vi "Treat Command.vi"(8 "error in (no error)":errorcluster, 11 "Channel in":refnum<class "Channel.lvclass">) -> (0 "error out":errorcluster, 3 "Channel out":refnum<class "Channel.lvclass">)   [LabVIEW 2018, in "Channel.lvclass"]
uses:
  Channel.lvclass
  Channel.lvclass/Channel.ctl
  TCS_ACS/TCS.lvclass/TCS.ctl
  Simulated_CCD_Camera/Simulated_CCD_Camera.lvclass/Simulated_CCD_Camera.ctl
  State Machine/State Machine.lvclass
  Simulated_CCD_Camera/Simulated_CCD_Camera.lvclass
  RxTx/RxTx.lvclass
  TCS_ACS/TCS.lvclass
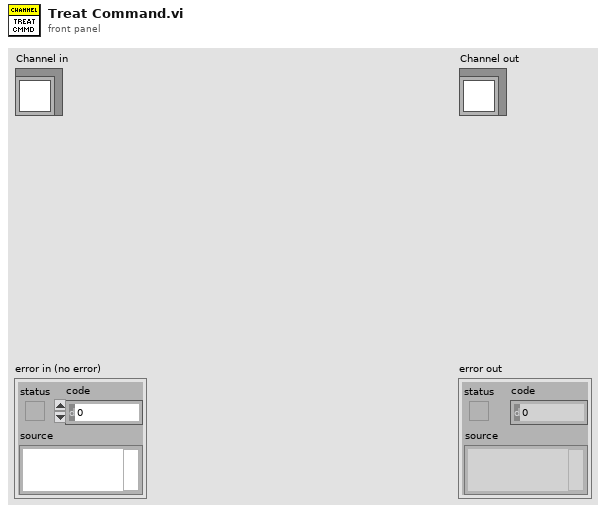
[diagram p1: front panel]
types:
  T1 = cluster{"CUBE_EXPOSURE_TIME":sgl, "CUBES_DONE":u16, "LAST_IMAGE_NAME":string, "DISK_SPACE":u16, "FRAMES_DONE":u16, "CCD_STATUS":string, "CURRENT_TEMPERATURE":i16, "TEMPERATURE_STATUS":string, "FRAME_EXPOSURE_TIME":dbl, "CCD_POWER_STATUS":bool, "SERIAL_NUMBER":u16, "ACQUIRING":bool}
  T2 = cluster{"COOLER_POWER_STATUS":u16, "TEMP":i32, "EXPTIME":sgl, "#FRAMES":u32, "#CUBES":u32}
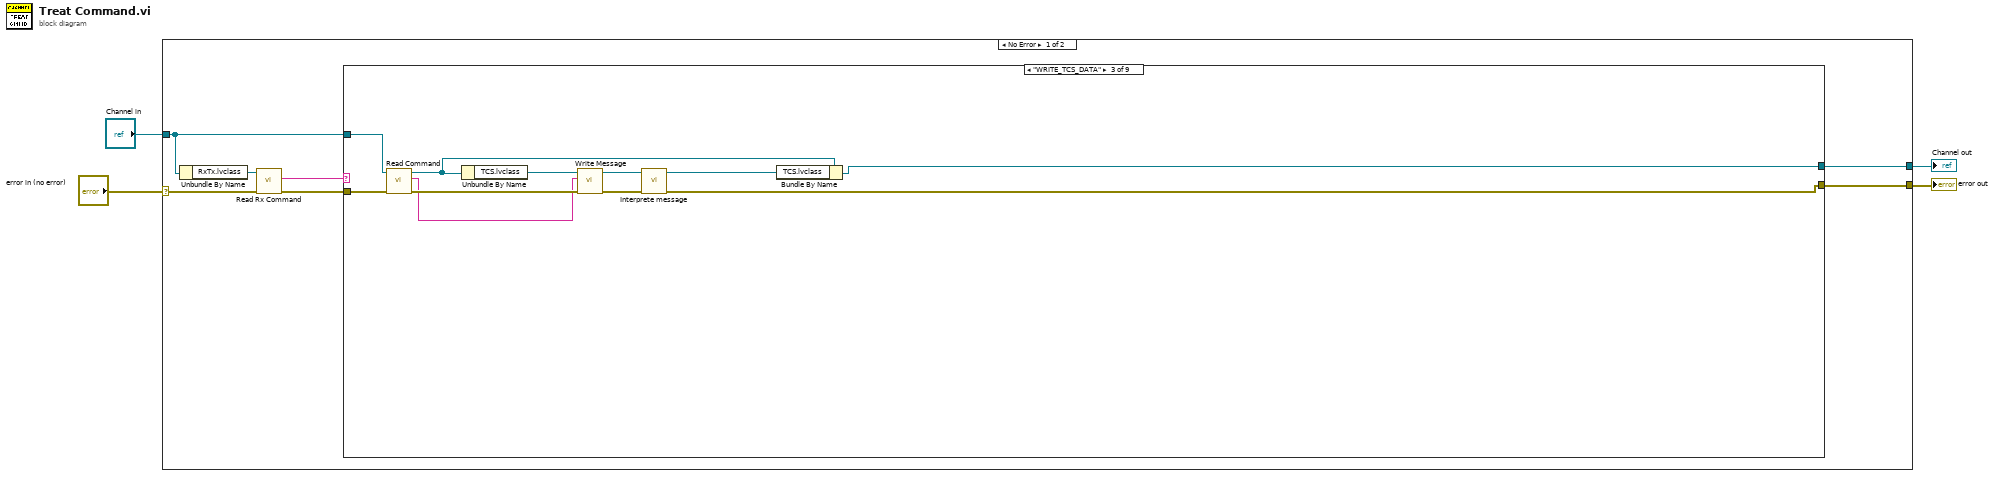
[diagram p0: block diagram]
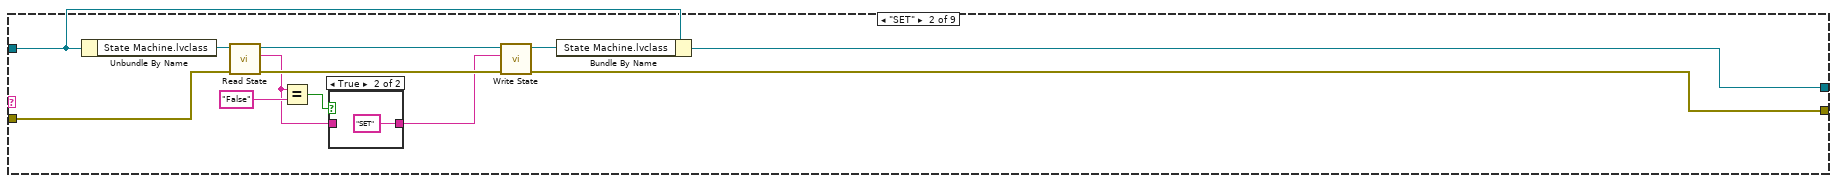
[diagram p3: hidden frame]
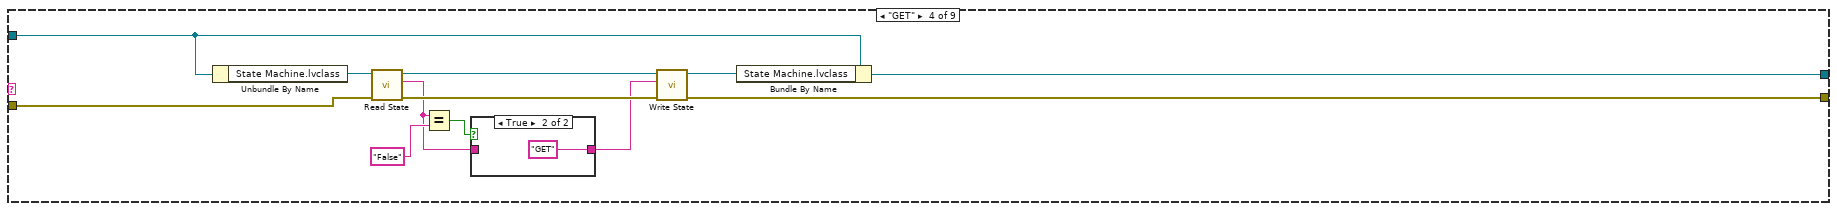
[diagram p5: hidden frame]
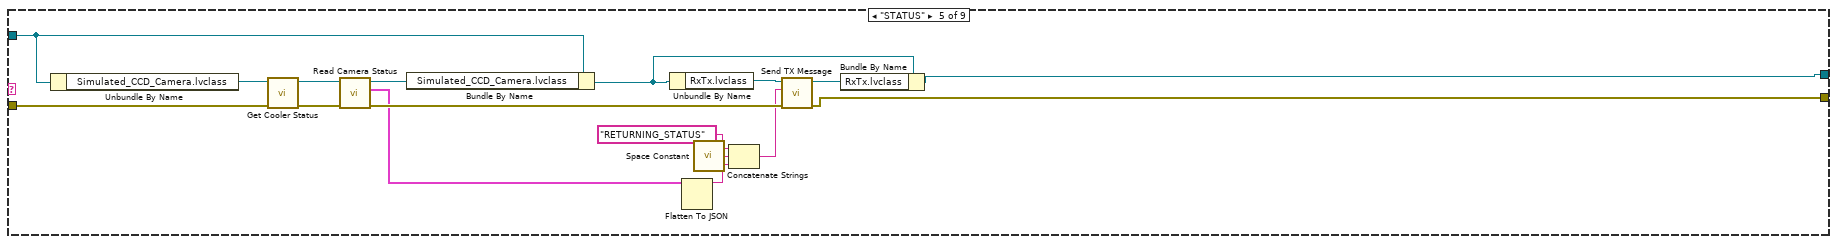
[diagram p7: hidden frame]
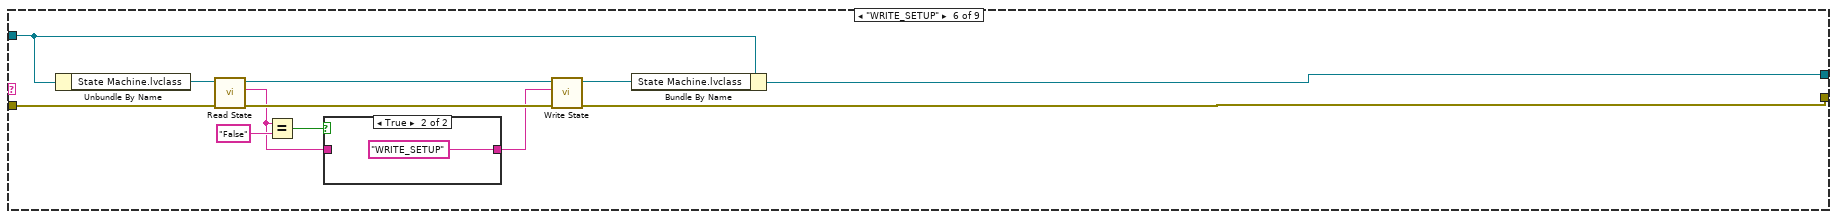
[diagram p8: hidden frame]
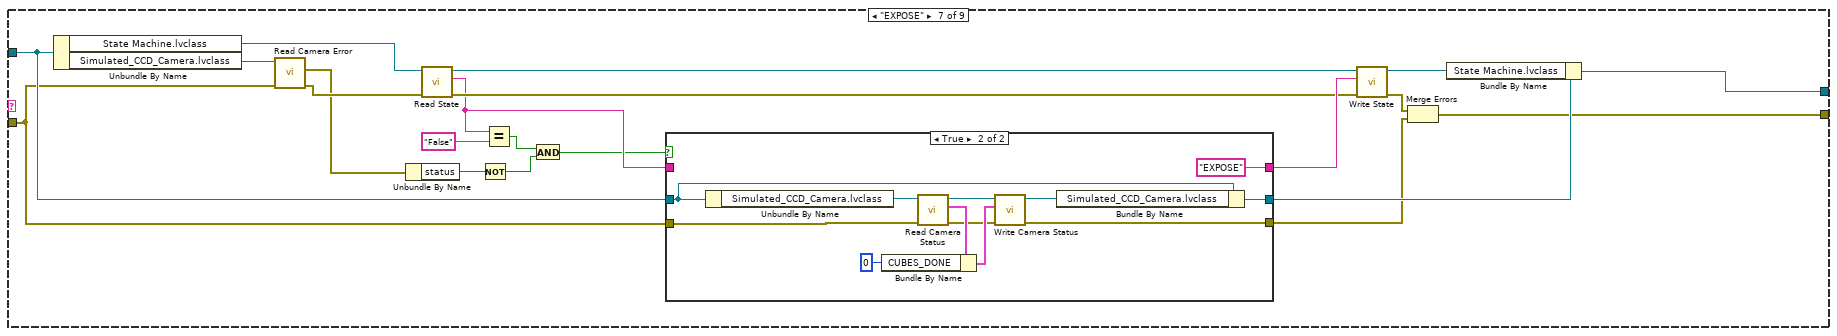
[diagram p10: hidden frame]
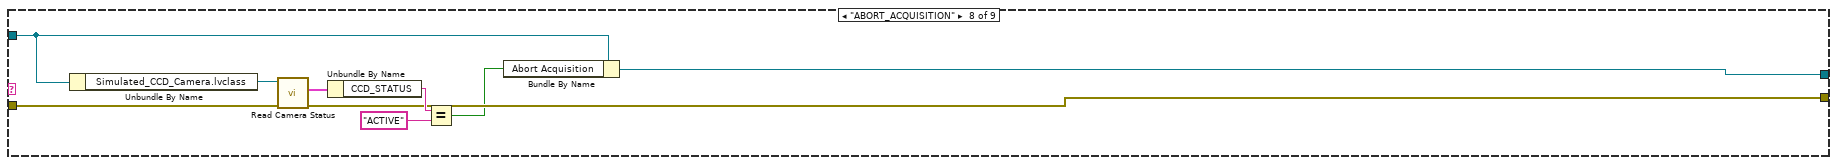
[diagram p12: hidden frame]
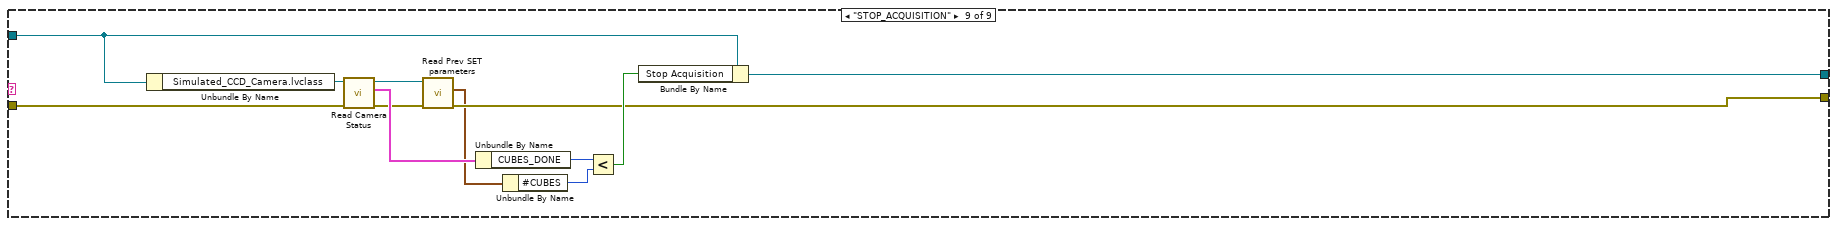
[diagram p13: hidden frame]
diagram:
  n1 = case shown="No Error" "error in (no error)" {
    selector: "error in (no error)" -> [w10 w142]
    tunnel: [w5 w142] -> w3
    tunnel: [w7 w141] -> w1
    tunnel: "Channel in" -> [w8 w141]
    frame No Error {
      n2 = Unbundle By Name(w8) -> ("RxTx.lvclass"=w11:refnum<class "RxTx.lvclass">)
      n3 = call "Read Rx Command.vi"("error in (no error)"=w10, "RxTx in"=w11) -> ("error out"=w6:errorcluster, "Rx Command"=w9:string)  [unwired: 7 in, 1 out]
      n4 = case shown="\"WRITE_TCS_DATA\"" w9 {
        tunnel: w8 -> [w13 w17 w37 w41 w69 w70 w98 w128 w138]
        tunnel: [w13 w14 w32 w40 w54 w76 w103 w127 w140] -> w7
        tunnel: w6 -> [w12 w16 w38 w42 w63 w74 w90 w122 w131]
        tunnel: [w12 w15 w28 w39 w53 w72 w96 w123 w134] -> w5
        frame "False", Default {
        }
        frame "SET" {
          n5 = Unbundle By Name(w17) -> ("State Machine.lvclass"=w23:refnum<class "State Machine.lvclass">)
          n6 = call-dynamic "Read State.vi"("error in (no error)"=w16, "State Machine in"=w23) -> ("error out"=w24:errorcluster, "State"=w19:string, "State Machine out"=w20:refnum<class "State Machine.lvclass">)  [unwired: 7 in]
          n7 = Equal?(x=w19, y="False") -> (x = y?=w18:bool)
          n8 = case shown="True" w18 {
            tunnel: [w26 "SET"] -> w22
            tunnel: w19 -> [w26 _]
            frame False {
            }
            frame True {
            }
          }
          n9 = call-dynamic "Write State.vi"("error in (no error)"=w24, "State"=w22, "State Machine in"=w20) -> ("error out"=w15:errorcluster, "State Machine out"=w25:refnum<class "State Machine.lvclass">)  [unwired: 7 in]
          n10 = Bundle By Name(cluster=w17, "State Machine.lvclass"=w25) -> (w14:refnum<class "Channel.lvclass">)
        }
        frame "WRITE_TCS_DATA" {
          n11 = call "Read Command.vi"("error in (no error)"=w38, "Channel in"=w37) -> ("error out"=w35:errorcluster, "Message"=w34:string, "Channel out"=w33:refnum<class "Channel.lvclass">)  [unwired: 7 in]
          n12 = Unbundle By Name(w33) -> ("TCS.lvclass"=w36:refnum<class "TCS.lvclass">)
          n13 = call "Write Message.vi"("error in (no error)"=w35, "Message"=w34, "TCS_ACS in"=w36) -> ("error out"=w29:errorcluster, "TCS_ACS out"=w31:refnum<class "TCS.lvclass">)  [unwired: 7 in]
          n14 = call "Interprete message.vi"("error in (no error)"=w29, "TCS_ACS in"=w31) -> ("error out"=w28:errorcluster, "TCS_ACS out"=w30:refnum<class "TCS.lvclass">)  [unwired: 8 in]
          n15 = Bundle By Name(cluster=w33, "TCS.lvclass"=w30) -> (w32:refnum<class "Channel.lvclass">)
        }
        frame "GET" {
          n16 = Unbundle By Name(w41) -> ("State Machine.lvclass"=w48:refnum<class "State Machine.lvclass">)
          n17 = call-dynamic "Read State.vi"("error in (no error)"=w42, "State Machine in"=w48) -> ("error out"=w49:errorcluster, "State"=w44:string, "State Machine out"=w45:refnum<class "State Machine.lvclass">)  [unwired: 7 in]
          n18 = Equal?(x=w44, y="False") -> (x = y?=w43:bool)
          n19 = case shown="True" w43 {
            tunnel: [w51 "GET"] -> w47
            tunnel: w44 -> [w51 _]
            frame False {
            }
            frame True {
            }
          }
          n20 = call-dynamic "Write State.vi"("error in (no error)"=w49, "State"=w47, "State Machine in"=w45) -> ("error out"=w39:errorcluster, "State Machine out"=w50:refnum<class "State Machine.lvclass">)  [unwired: 7 in]
          n21 = Bundle By Name(cluster=w41, "State Machine.lvclass"=w50) -> (w40:refnum<class "Channel.lvclass">)
        }
        frame "STATUS" {
          n22 = Unbundle By Name(w69) -> ("Simulated_CCD_Camera.lvclass"=w65:refnum<class "Simulated_CCD_Camera.lvclass">)
          n23 = call-dynamic "Get Cooler Status.vi"("error in (no error)"=w63, "CCDCamera in"=w65) -> ("error out"=w66:errorcluster, "CCDCamera out"=w67:refnum<class "Simulated_CCD_Camera.lvclass">)  [unwired: 8 in]
          n24 = call "Read Camera Status.vi"("error in (no error)"=w66, "CCDCamera in"=w67) -> ("error out"=w60:errorcluster, "Camera Status"=w56:T1, "CCDCamera out"=w64:refnum<class "Simulated_CCD_Camera.lvclass">)  [unwired: 7 in]
          n25 = Bundle By Name(cluster=w69, "Simulated_CCD_Camera.lvclass"=w64) -> (w68:refnum<class "Channel.lvclass">)
          n26 = Unbundle By Name(w68) -> ("RxTx.lvclass"=w62:refnum<class "RxTx.lvclass">)
          n27 = Flatten To JSON(anything=w56) -> (JSON string=w57:string)  [unwired: 2 in, 1 out]
          n28 = call <vilib>:"Space Constant.vi"() -> ("String"=w58:string)
          n29 = Concatenate Strings("RETURNING_STATUS", w58, w57) -> (w55:string)
          n30 = call "Send TX Message.vi"("error in (no error)"=w60, "element"=w55, "RxTx in"=w62) -> ("error out"=w53:errorcluster, "RxTx out"=w61:refnum<class "RxTx.lvclass">)  [unwired: 7 in]
          n31 = Bundle By Name(cluster=w68, "RxTx.lvclass"=w61) -> (w54:refnum<class "Channel.lvclass">)
        }
        frame "WRITE_SETUP" {
          n32 = Unbundle By Name(w70) -> ("State Machine.lvclass"=w79:refnum<class "State Machine.lvclass">)
          n33 = call-dynamic "Read State.vi"("error in (no error)"=w74, "State Machine in"=w79) -> ("error out"=w80:errorcluster, "State"=w71:string, "State Machine out"=w77:refnum<class "State Machine.lvclass">)  [unwired: 7 in]
          n34 = Equal?(x=w71, y="False") -> (x = y?=w75:bool)
          n35 = case shown="True" w75 {
            tunnel: [w82 "WRITE_SETUP"] -> w73
            tunnel: w71 -> [w82 _]
            frame False {
            }
            frame True {
            }
          }
          n36 = call-dynamic "Write State.vi"("error in (no error)"=w80, "State"=w73, "State Machine in"=w77) -> ("error out"=w72:errorcluster, "State Machine out"=w81:refnum<class "State Machine.lvclass">)  [unwired: 7 in]
          n37 = Bundle By Name(cluster=w70, "State Machine.lvclass"=w81) -> (w76:refnum<class "Channel.lvclass">)
        }
        frame "EXPOSE" {
          n38 = Unbundle By Name(w98) -> ("State Machine.lvclass"=w102:refnum<class "State Machine.lvclass">, "Simulated_CCD_Camera.lvclass"=w93:refnum<class "Simulated_CCD_Camera.lvclass">)
          n39 = call "Read Camera Error.vi"("error in (no error)"=w90, "Simulated_CCD_Camera in"=w93) -> ("error out"=w92:errorcluster, "Camera Error"=w89:errorcluster)  [unwired: 7 in, 1 out]
          n40 = Unbundle By Name(w89) -> ("status"=w87:bool)
          n41 = call-dynamic "Read State.vi"("error in (no error)"=w92, "State Machine in"=w102) -> ("error out"=w91:errorcluster, "State"=w88:string, "State Machine out"=w99:refnum<class "State Machine.lvclass">)  [unwired: 7 in]
          n42 = Not(x=w87) -> (.not. x?=w85:bool)
          n43 = Equal?(x=w88, y="False") -> (x = y?=w86:bool)
          n44 = And(x=w86, y=w85) -> (x .and. y?=w84:bool)
          n45 = case shown="True" w84 {
            tunnel: [w105 "EXPOSE"] -> w101
            tunnel: w98 -> [w107 w118]
            tunnel: w90 -> [w106 w117]
            tunnel: [w107 w116] -> w97
            tunnel: [w106 w115] -> w94
            tunnel: w88 -> [w105 _]
            frame False {
            }
            frame True {
              n46 = Unbundle By Name(w118) -> ("Simulated_CCD_Camera.lvclass"=w109:refnum<class "Simulated_CCD_Camera.lvclass">)
              n47 = call "Read Camera Status.vi"("error in (no error)"=w117, "CCDCamera in"=w109) -> ("error out"=w110:errorcluster, "Camera Status"=w112:T1, "CCDCamera out"=w113:refnum<class "Simulated_CCD_Camera.lvclass">)  [unwired: 7 in]
              n48 = Bundle By Name(cluster=w112, "CUBES_DONE"=u16 0) -> (w111:T1)
              n49 = call "Write Camera Status.vi"("error in (no error)"=w110, "Camera Status"=w111, "CCDCamera in"=w113) -> ("error out"=w115:errorcluster, "CCDCamera out"=w108:refnum<class "Simulated_CCD_Camera.lvclass">)  [unwired: 7 in]
              n50 = Bundle By Name(cluster=w118, "Simulated_CCD_Camera.lvclass"=w108) -> (w116:refnum<class "Channel.lvclass">)
            }
          }
          n51 = call-dynamic "Write State.vi"("error in (no error)"=w91, "State"=w101, "State Machine in"=w99) -> ("error out"=w95:errorcluster, "State Machine out"=w104:refnum<class "State Machine.lvclass">)  [unwired: 7 in]
          n52 = Merge Errors(w95, w94) -> (w96:errorcluster)
          n53 = Bundle By Name(cluster=w97, "State Machine.lvclass"=w104) -> (w103:refnum<class "Channel.lvclass">)
        }
        frame "ABORT_ACQUISITION" {
          n54 = Unbundle By Name(w128) -> ("Simulated_CCD_Camera.lvclass"=w121:refnum<class "Simulated_CCD_Camera.lvclass">)
          n55 = call "Read Camera Status.vi"("error in (no error)"=w122, "CCDCamera in"=w121) -> ("error out"=w123:errorcluster, "Camera Status"=w126:T1)  [unwired: 7 in, 1 out]
          n56 = Unbundle By Name(w126) -> ("CCD_STATUS"=w125:string)
          n57 = Equal?(x=w125, y="ACTIVE") -> (x = y?=w120:bool)
          n58 = Bundle By Name(cluster=w128, "Abort Acquisition"=w120) -> (w127:refnum<class "Channel.lvclass">)
        }
        frame "STOP_ACQUISITION" {
          n59 = Unbundle By Name(w138) -> ("Simulated_CCD_Camera.lvclass"=w132:refnum<class "Simulated_CCD_Camera.lvclass">)
          n60 = call "Read Camera Status.vi"("error in (no error)"=w131, "CCDCamera in"=w132) -> ("error out"=w130:errorcluster, "Camera Status"=w137:T1, "CCDCamera out"=w129:refnum<class "Simulated_CCD_Camera.lvclass">)  [unwired: 7 in]
          n61 = call-dynamic "Read Prev SET parameters.vi"("error in (no error)"=w130, "Simulated_CCD_Camera in"=w129) -> ("error out"=w134:errorcluster, "Prev SET parameters"=w133:T2)  [unwired: 7 in, 1 out]
          n62 = Unbundle By Name(w137) -> ("CUBES_DONE"=w136:u16)
          n63 = Unbundle By Name(w133) -> ("#CUBES"=w135:u32)
          n64 = Less?(x=w136, y=w135) -> (x < y?=w139:bool)
          n65 = Bundle By Name(cluster=w138, "Stop Acquisition"=w139) -> (w140:refnum<class "Channel.lvclass">)
        }
      }
    }
    frame Error {
    }
  }
  "error out" <- w3
  "Channel out" <- w1
